vi "ReadI16.vi"(11 "Address":u32) -> (3 "Data":i16)   [LabVIEW 2018]
uses:
  <vilib>/rvi/Memory/Memory_Emulation/nirvimemoryFastEmulation.vi
  <vilib>/rvi/Memory/Memory_Emulation/nirvimemoryEmulation.vi
  <vilib>/rvi/Emulation/niFpgaEmulationIsFPGAContextNoSignature.vi
  <vilib>/rvi/DataTransferAndStorage/Container/Common/niFpgaContainerGetUniqueNameForEmu.vi
  <vilib>/rvi/Emulation/niFpgaProcessEmulError.vi
  <vilib>/rvi/Emulation/niFpgaSctlEmulationGetInTimedLoop.vi
  <vilib>/rvi/errors/nirviReportUnexpectedCaseInternalError (U32).vi
  <vilib>/rvi/DataTransferAndStorage/Container/Common/niFpgaContainerExecOnDevCompGetState.vi
  <vilib>/rvi/Memory/Memory_Emulation/niFpgaMemoryEmulationCacheClearOnFirstRun.vi
  <vilib>/rvi/Memory/Memory_Emulation/nirvimemoryEmulationManagerCache_MakeExclusive.vi
  <vilib>/rvi/Memory/Memory_Emulation/niFpgaMemoryEmulationValidateCache.vi
  <vilib>/rvi/Memory/Memory_Emulation/nirvimemoryEmulationManagerCache_InsertValue.vi
  <vilib>/Utility/error.llb/Clear Errors.vi
  <vilib>/rvi/Memory/Memory_Emulation/nirvimemoryEmulationManagerCache_ReleaseExclusive.vi
  <vilib>/rvi/Memory/Memory_Emulation/nirvimemoryEmulationManagerCache_GetValue.vi
  <vilib>/rvi/Memory/Memory_Emulation/nirvimemoryEmulationManagerCache_SetValue.vi
  <vilib>/rvi/Emulation/niFpgaSctlEmulationResourceMgr.vi
  <vilib>/rvi/DataTransferAndStorage/Container/XNode/niFpgaContainer.xnode
  <vilib>/rvi/Memory/Memory_Emulation/niFpgaMemoryEmulationRefIn.vi
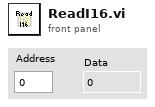
[diagram p1: front panel]
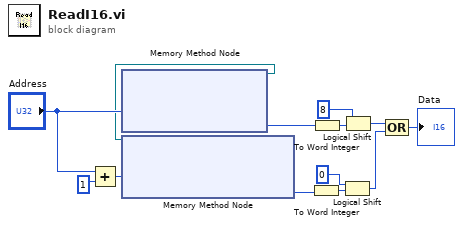
[diagram p0: block diagram]
diagram:
  n1 = Add(x="Address", y=u32 1) -> (x+y=w3:u32)
  n2 = xnode ("Memory Method Node")("Address"="Address") -> ("Data"=w13:u8, "Memory Out"=w1:refnum<k21>)  [unwired: 1 in]
  n3 = xnode ("Memory Method Node")("Address"=w3, "Memory In"=w1) -> ("Data"=w9:u8)  [unwired: 1 out]
  n4 = To Word Integer(number=w9) -> (16bit integer=w10:i16)
  n5 = To Word Integer(number=w13) -> (16bit integer=w12:i16)
  n6 = Logical Shift(y=i16 0, x=w10) -> (x << y=w7:i16)
  n7 = Logical Shift(y=i16 8, x=w12) -> (x << y=w2:i16)
  n8 = Compound Arithmetic op=OR(w2, w7) -> (→"Data":i16)
